vi "BestFitFOAW.vi"(0 "y_k":dbl, 1 "d":dbl, 2 "T":dbl, 3 "n_max":i32=10) -> (7 "vel estimation":dbl, 9 "window length":i32)   [LabVIEW 2019]
panel:
  in  "found":bool
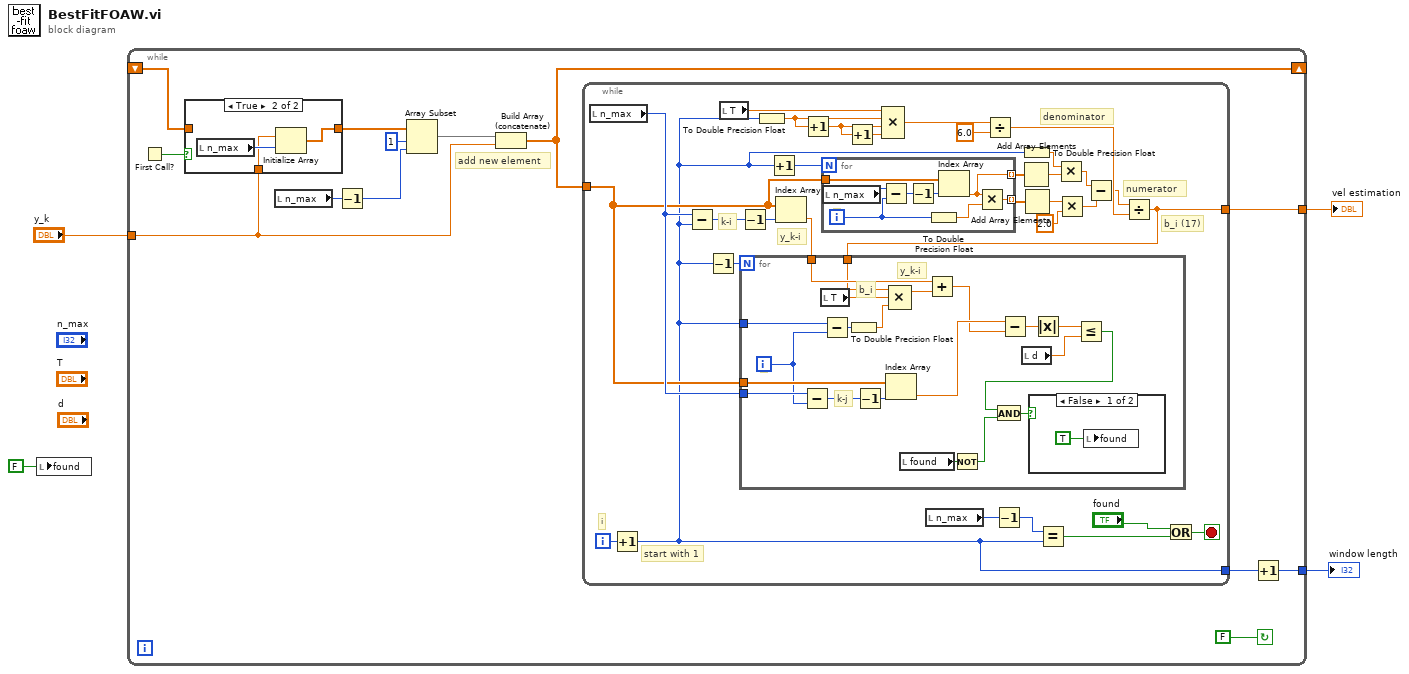
[diagram p0: block diagram]
diagram:
  n1 = local write "found"(FALSE ("found")) -> ()
  n2 = while {
    tunnel: "y_k" -> [w5]
    tunnel: [w16] -> w2
    shift-right: [w9] -> _
    shift-left: _ -> [w11]
    tunnel: [w7] -> w1
    stop <- FALSE continue-if-true
    # "add new element"
    n3 = First Call?() -> (First Call?: T/F=w10:bool)
    n4 = case shown="True" w10 {
      tunnel: [w18 w20] -> w6
      tunnel: w11 -> [w18 _]
      tunnel: w5 -> [_ w19]
      frame False {
      }
      frame True {
        n5 = local read "n_max"() -> (w21:i32)
        n6 = Initialize Array(w19, w21) -> (w20:dbl[])
      }
    }
    n7 = local read "n_max"() -> (w14:i32)
    n8 = Decrement(x=w14) -> (x-1=w13:i32)
    n9 = Array Subset(array=w6, index=1, length=w13) -> (w12:dbl[])
    n10 = Build Array (concatenate)(w12, w5) -> (w9:dbl[])
    n11 = while {
      tunnel: w9 -> [w33]
      tunnel: [w44] -> w16
      tunnel: [w29] -> w8
      i -> [w47]
      stop <- w50 stop-if-true
      # "numerator"
      # "b_i (17)"
      # "i"
      # "start with 1"
      # "y_k-i"
      # "denominator"
      # "k-i"
      n12 = local read "n_max"() -> (w45:i32)
      n13 = Increment(x=w47) -> (x+1=w29:i32)
      n14 = Subtract(x=w45, y=w29) -> (x-y=w52:i32)
      n15 = Decrement(x=w29) -> (x-1=w46:i32)
      n16 = local read "T"() -> (w42:dbl)
      n17 = Decrement(x=w52) -> (x-1=w35:i32)
      n18 = To Double Precision Float(number=w29) -> (double precision float=w41:dbl)
      n19 = Increment(x=w29) -> (x+1=w23:i32)
      n20 = Index Array(array=w33, index=w35) -> (element=w36:dbl)
      n21 = Increment(x=w41) -> (x+1=w40:dbl)
      n22 = for {
        N: w23 -> [_]
        tunnel: w33 -> [w60]
        tunnel: [w58] -> w32 mode=indexing
        tunnel: [w57] -> w31 mode=indexing
        i -> [w55]
        # "j"
        n23 = local read "n_max"() -> (w56:i32)
        n24 = Subtract(x=w56, y=w55) -> (x-y=w54:i32)
        n25 = Decrement(x=w54) -> (x-1=w53:i32)
        n26 = To Double Precision Float(number=w55) -> (double precision float=w59:dbl)
        n27 = Index Array(array=w60, index=w53) -> (element=w57:dbl)
        n28 = Multiply(x=w57, y=w59) -> (x*y=w58:dbl)
      }
      n29 = Increment(x=w40) -> (x+1=w39:dbl)
      n30 = Compound Arithmetic op=MULTIPLY(w42, w41, w40, w39) -> (w22:dbl)
      n31 = local read "n_max"() -> (w49:i32)
      n32 = Divide(x=w22, y=6.0) -> (x/y=w38:dbl)
      n33 = Decrement(x=w49) -> (x-1=w43:i32)
      n34 = Add Array Elements(numeric array=w31) -> (sum=w30:dbl)
      n35 = To Double Precision Float(number=w29) -> (double precision float=w28:dbl)
      n36 = Add Array Elements(numeric array=w32) -> (sum=w34:dbl)
      n37 = Equal?(x=w43, y=w29) -> (x = y?=w48:bool)
      n38 = Multiply(x=w28, y=w30) -> (x*y=w25:dbl)
      n39 = Multiply(x=w34, y=2.0) -> (x*y=w26:dbl)
      n40 = Subtract(x=w25, y=w26) -> (x-y=w24:dbl)
      n41 = Divide(x=w24, y=w38) -> (x/y=w44:dbl)
      n42 = for {
        N: w46 -> [_]
        tunnel: w33 -> [w71]
        tunnel: w36 -> [w78]
        tunnel: w44 -> [w75]
        tunnel: w29 -> [w74]
        tunnel: w45 -> [w69]
        i -> [w68]
        # "b_i"
        # "y_k-i"
        # "k-j"
        # "j"
        n43 = Subtract(x=w69, y=w68) -> (x-y=w70:i32)
        n44 = local read "T"() -> (w76:dbl)
        n45 = Subtract(x=w74, y=w68) -> (x-y=w73:i32)
        n46 = To Double Precision Float(number=w73) -> (double precision float=w72:dbl)
        n47 = Decrement(x=w70) -> (x-1=w61:i32)
        n48 = Index Array(array=w71, index=w61) -> (element=w67:dbl)
        n49 = Compound Arithmetic op=MULTIPLY(w75, w76, w72) -> (w77:dbl)
        n50 = local read "found"() -> (w80:bool)
        n51 = Add(x=w78, y=w77) -> (x+y=w66:dbl)
        n52 = Not(x=w80) -> (.not. x?=w79:bool)
        n53 = Subtract(x=w67, y=w66) -> (x-y=w65:dbl)
        n54 = local read "d"() -> (w63:dbl)
        n55 = Absolute Value(x=w65) -> (abs(x)=w64:dbl)
        n56 = Less Or Equal?(x=w64, y=w63) -> (x <= y?=w62:bool)
        n57 = And(x=w62, y=w79) -> (x .and. y?=w81:bool)
        n58 = case shown="False" w81 {
          frame False {
            n59 = local write "found"(TRUE ("found")) -> ()
          }
          frame True {
          }
        }
      }
      n60 = Or(x="found", y=w48) -> (x .or. y?=w50:bool)
    }
    n61 = Increment(x=w8) -> (x+1=w7:i32)
  }
  "vel estimation" <- w2
  "window length" <- w1
